vi "PH_Beamline_Common.set PA Aperture Selector.vi"(2 "CtlRef":refnum<vi>, 3 "State":T1 items=["unknown", "Position I", "Position II", "Position III", "Position IV", "moving"], 4 "no link":bool, 5 "error in (no error)":errorcluster) -> (19 "error out":errorcluster)   [LabVIEW 2014, in "PH_Beamline_Common.lvlib"]
uses:
  PH_Beamline_Common.lvlib
  PH_Motion/PH_4_Pos_Selector/PH_4_Pos_Selector.Position Selector.ctl
  PH_Common/PH_Common.lvlib
  PH_Motion/PH_4_Pos_Selector/PH_4_Pos_Selector.lvlib
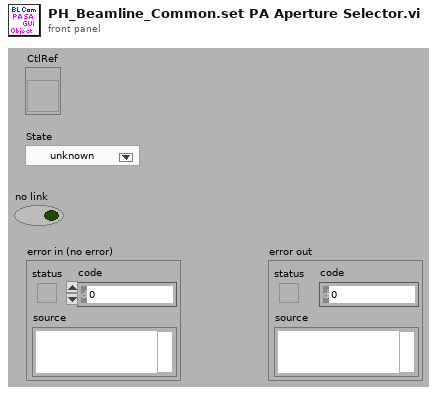
[diagram p1: front panel]
types:
  T1 = typedef "PH_4_Pos_Selector.lvlib/PH_4_Pos_Selector.Position Selector.ctl" = u16
  T2 = cluster{"left":i16, "top":i16, "right":i16, "bottom":i16}[]
  T3 = cluster{"left":i16, "top":i16, "right":i16, "bottom":i16}
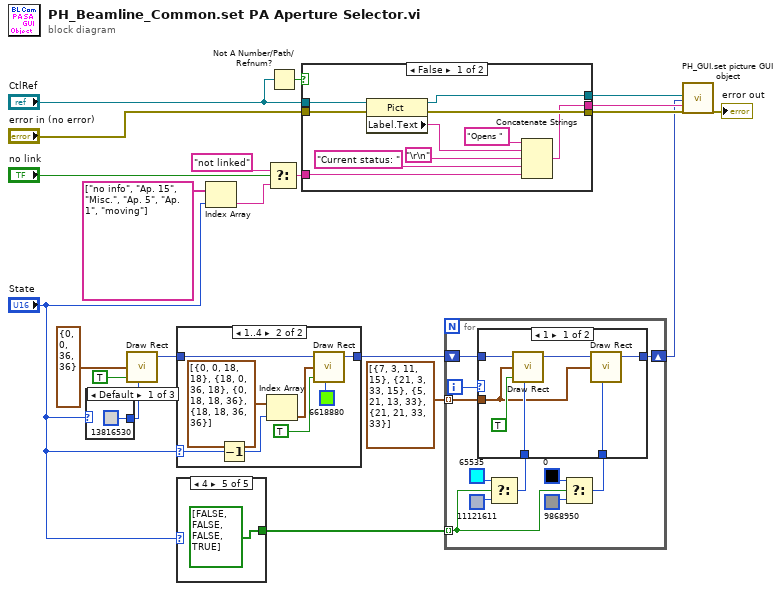
[diagram p0: block diagram]
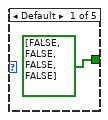
[diagram p2: hidden frame]
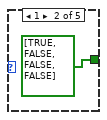
[diagram p3: hidden frame]
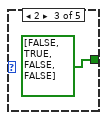
[diagram p4: hidden frame]
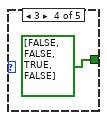
[diagram p5: hidden frame]
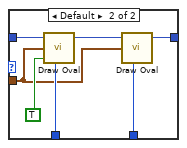
[diagram p6: hidden frame]
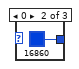
[diagram p8: hidden frame]
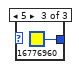
[diagram p9: hidden frame]
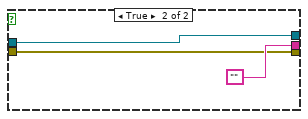
[diagram p10: hidden frame]
diagram:
  n1 = case shown="Default" "State" {
    tunnel: [u32 13816530 u32 16860 u32 16776960] -> w8
    frame Default {
    }
    frame 0 {
    }
    frame 5 {
    }
  }
  n2 = call <vilib>:"Draw Rect.vi"("rect"=T3 {"left"=0, "top"=0, "right"=36, "bottom"=36}, "fill?(F)"=TRUE, "color(black)"=w8) -> ("new picture"=w7:picture)  [unwired: 6 in]
  n3 = case shown="1..4" "State" {
    selector: "State" -> [_ w29]
    tunnel: w7 -> [w25 w33]
    tunnel: [w25 w28] -> w5
    frame Default {
    }
    frame 1..4 {
      n4 = Decrement(x=w29) -> (x-1=w26:T1)
      n5 = Index Array(array=T2 [{"left"=0, "top"=0, "right"=18, "bottom"=18}, {"left"=18, "top"=0, "right"=36, "bottom"=18}, {"left"=0, "top"=18, "right"=18, "bottom"=36}, {"left"=18, "top"=18, "right"=36, "bottom"=36}], index=w26) -> (element=w30:T3)
      n6 = call <vilib>:"Draw Rect.vi"("picture"=w33, "rect"=w30, "fill?(F)"=TRUE, "color(black)"=u32 6618880) -> ("new picture"=w28:picture)  [unwired: 5 in]
    }
  }
  n7 = case shown="4" "State" {
    tunnel: [bool[] [FALSE, FALSE, FALSE, FALSE] bool[] [TRUE, FALSE, FALSE, FALSE] bool[] [FALSE, TRUE, FALSE, FALSE] bool[] [FALSE, FALSE, TRUE, FALSE] bool[] [FALSE, FALSE, FALSE, TRUE]] -> w2
    frame Default {
    }
    frame 1 {
    }
    frame 2 {
    }
    frame 3 {
    }
    frame 4 {
    }
  }
  n8 = Index Array(array=string[] ["no info", "Ap. 15", "Misc.", "Ap. 5", "Ap. 1", "moving"], index="State") -> (element=w10:string)
  n9 = Select(t="not linked" ("string"), s="no link", f=w10) -> (s? t:f=w13:string)
  n10 = Not A Number/Path/Refnum?(number/path/refnum="CtlRef") -> (NaN/Path/Refnum?=w15:bool)
  n11 = case shown="False" w15 {
    tunnel: "CtlRef" -> [w44 w51]
    tunnel: "error in (no error)" -> [w43 w49]
    tunnel: [w42 w49] -> w18
    tunnel: w13 -> [w41 _]
    tunnel: [w40 ""] -> w17
    tunnel: [w39 w51] -> w16
    frame False {
      n12 = property class="Pict"(reference=w44, error in=w43) -> (reference out=w39:refnum<vi>, error out=w42:errorcluster, "Label.Text"=w47:string)
      n13 = Concatenate Strings("Opens " ("string"), w47, "\r\n", "Current status: " ("string"), w41) -> (w40:string)
    }
    frame True {
    }
  }
  n14 = for {
    shift-right: [w61] -> w3
    shift-left: w5 -> [w62]
    tunnel: T2 [{"left"=7, "top"=3, "right"=11, "bottom"=15}, {"left"=21, "top"=3, "right"=33, "bottom"=15}, {"left"=5, "top"=21, "right"=13, "bottom"=33}, {"left"=21, "top"=21, "right"=33, "bottom"=33}] -> [w60] mode=indexing
    tunnel: w2 -> [w53] mode=indexing
    i -> [w59]
    n15 = Select(t=u32 65535 ("color(black)"), s=w53, f=u32 11121611) -> (s? t:f=w56:u32)
    n16 = Select(t=u32 0 ("color(black)"), s=w53, f=u32 9868950) -> (s? t:f=w52:u32)
    n17 = case shown="1" w59 {
      tunnel: w62 -> [w69 w76]
      tunnel: w56 -> [w68 w74]
      tunnel: [w64 w72] -> w61
      tunnel: w60 -> [w63 w71]
      tunnel: w52 -> [w66 w70]
      frame 1 {
        n18 = call <vilib>:"Draw Rect.vi"("picture"=w69, "rect"=w63, "fill?(F)"=TRUE, "color(black)"=w68) -> ("new picture"=w65:picture)  [unwired: 5 in]
        n19 = call <vilib>:"Draw Rect.vi"("picture"=w65, "rect"=w63, "color(black)"=w66) -> ("new picture"=w64:picture)  [unwired: 6 in]
      }
      frame Default {
        n20 = call <vilib>:"Draw Oval.vi"("picture"=w76, "rect"=w71, "fill?(F)"=TRUE, "color(black)"=w74) -> ("new picture"=w73:picture)  [unwired: 5 in]
        n21 = call <vilib>:"Draw Oval.vi"("picture"=w73, "rect"=w71, "color(black)"=w70) -> ("new picture"=w72:picture)  [unwired: 6 in]
      }
    }
  }
  n22 = call "PH_GUI.set picture GUI object.vi"("CtlRef"=w16, "Picture"=w3, "Tip Strip (\"\")"=w17, "error in (no error)"=w18) -> ("error out"=→"error out":errorcluster)  [unwired: 15 in]
